vi "HB_ImaqGrab.vi"() -> ()   [LabVIEW 2009, in "HB_IMAQ_Examples.lvlib"]
uses:
  lib.lib/HGF_LVC/HGF_IMAQ/HGF_IMAQFactory/HGF_IMAQFactory.lvclass
  lib.lib/HGF_LVC/HGF_IMAQ/HGF_IMAQDevice/HGF_IMAQDevice.lvclass
  HB_IMAQ_Examples.lvlib
  lib.lib/HGF_LVC/HGF_BaseClasses/HGF_Factory/HGF_Factory.lvclass
  lib.lib/HGF_LVC/HGF_DeviceBaseClasses/HGF_DeviceBase/HGF_DeviceBase.lvclass
  lib.lib/HGF_LVC/HGF_Auxiliary/HGF_Auxiliary.lvlib
panel:
  out "Acquired Buffer Number":u32
  out "iteration":i32
  out "Image":T1(plugin-control)
  in  "interval / ms":u32=100
  in  "stop":bool
  in  "Image Type":T2 items=["Grayscale (U8)", "Grayscale (I16)", "Grayscale (SGL)", "Complex (CSG)", "RGB (U32)", "HSL (U32)", "RGB (U64)", "Grayscale (U16)"]
  in  "cameraName":string="cam0"
  in  "imaqClassName":string="HGF_ImaqDx"
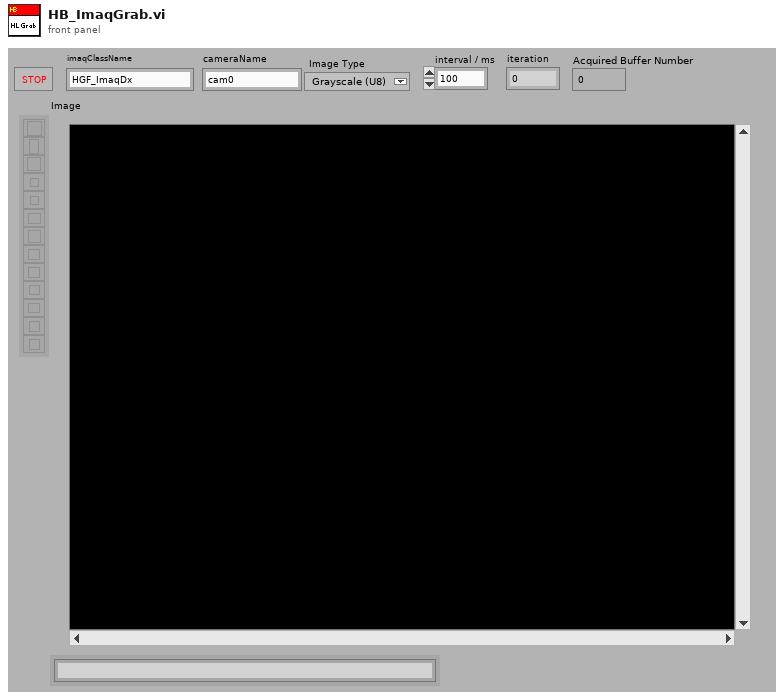
[diagram p1: front panel]
types:
  T1 = typedef "IMAQ Image.ctl" = refnum<image>
  T2 = typedef "Image Type" = u32
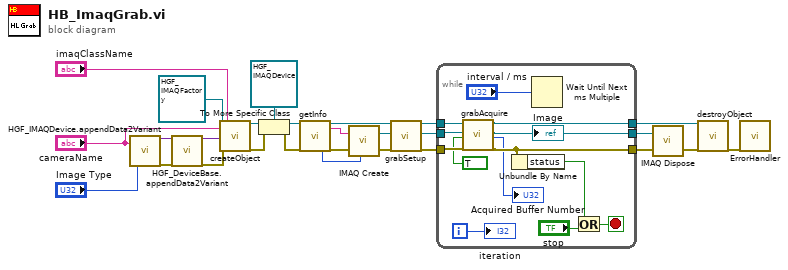
[diagram p0: block diagram]
diagram:
  n1 = call "HGF_IMAQDevice.appendData2Variant.vi"("cameraName"="cameraName", "imageType"="Image Type") -> ("dup initData"=w26:variant, "error out"=w25:errorcluster)  [unwired: 4 in, 12 out]
  n2 = call "HGF_DeviceBase.appendData2Variant.vi"("initData"=w26, "error in (no error)"=w25) -> ("dup initData"=w23:variant, "error out"=w24:errorcluster)  [unwired: 16 out]
  n3 = call "createObject.vi"("HGF_Factory"=refnum<class "HGF_IMAQFactory.lvclass"> refnum ("HGF_IMAQ.lvlib:HGF_IMAQFactory.lvclass"), "objectName"="cameraName", "initializationData"=w23, "error in (no error)"=w24, "className"="imaqClassName") -> ("HGF_Object"=w20:refnum<class "HGF_Factory.lvclass">, "error out"=w19:errorcluster)  [unwired: 13 out]
  n4 = To More Specific Class(target class=refnum<class "HGF_IMAQDevice.lvclass"> refnum ("HGF_DeviceBaseClasses.lvlib:HGF_IMAQDevice.lvclass"), reference=w20, error in=w19) -> (specific class reference=w11:refnum<class "HGF_IMAQDevice.lvclass">, error out=w10:errorcluster)
  n5 = call "getInfo.vi"("HGF_IMAQDevice"=w11, "error in (no error)"=w10) -> ("imageType"=w5:T2, "dup HGF_IMAQDevice"=w4:refnum<class "HGF_IMAQDevice.lvclass">, "cameraName"=w7:string, "error out"=w9:errorcluster)  [unwired: 12 in, 2 out]
  n6 = call "IMAQ Create"("Image Name"=w7, "Image Type"=w5, "error in (no error)"=w9) -> ("New Image"=w17:T1, "error out"=w2:errorcluster)  [unwired: 1 in, 1 out]
  n7 = call "grabSetup.vi"("HGF_IMAQDevice"=w4, "error in (no error)"=w2) -> ("dup HGF_IMAQDevice"=w3:refnum<class "HGF_IMAQDevice.lvclass">, "error out"=w1:errorcluster)  [unwired: 16 in]
  n8 = while {
    tunnel: w3 -> [w34]
    tunnel: w1 -> [w33]
    tunnel: w17 -> [w32]
    tunnel: [w29] -> w16
    tunnel: [w30] -> w15
    tunnel: [w31] -> w13
    i -> [w35]
    stop <- w37 stop-if-true
    n9 = call "grabAcquire.vi"("HGF_IMAQDevice"=w34, "Image In"=w32, "Wait for Next Buffer? (Yes)"=TRUE, "error in (no error)"=w33) -> ("dup HGF_IMAQDevice"=w31:refnum<class "HGF_IMAQDevice.lvclass">, "Image Out"=w29:T1, "Acquired Buffer Number"=→"Acquired Buffer Number":u32, "error out"=w30:errorcluster)  [unwired: 12 in]
    "Image" <- w29
    n10 = Unbundle By Name(w30) -> ("status"=w39:bool)
    n11 = Wait Until Next ms Multiple(millisecond multiple="interval / ms") -> ()  [unwired: 1 out]
    n12 = Or(x=w39, y="stop") -> (x .or. y?=w37:bool)
    "iteration" <- w35
  }
  n13 = call "IMAQ Dispose"("Image"=w16, "error in (no error)"=w15) -> ("error out"=w14:errorcluster)  [unwired: 1 in, 3 out]
  n14 = call "destroyObject.vi"("HGF_Factory"=w13, "error in (no error)"=w14) -> ("error out"=w12:errorcluster)  [unwired: 17 out]
  n15 = call "ErrorHandler.vi"("error in (no error)"=w12) -> ()  [unwired: 6 in, 13 out]
